vi "MTMount_logEvent_heartbeat.vi"(8 "error in (no error)":errorcluster, 11 "logevent_heartbeat_Ctl":T1) -> (0 "error out":errorcluster, 2 "function return":i32, 3 "logevent_heartbeat_Ctl out":T1)   [LabVIEW 2018, in "SALLV_MTMount.lvlib"]
doc: "int MTMount_shm_logEvent_heartbeatLV(MTMount_logevent_heartbeatLV *logevent_heartbeat_Ctl );"
uses:
  SALLV_MTMount.lvlib
  DataTypes/logevent_heartbeat.ctl
  SALLV_MTMount.so
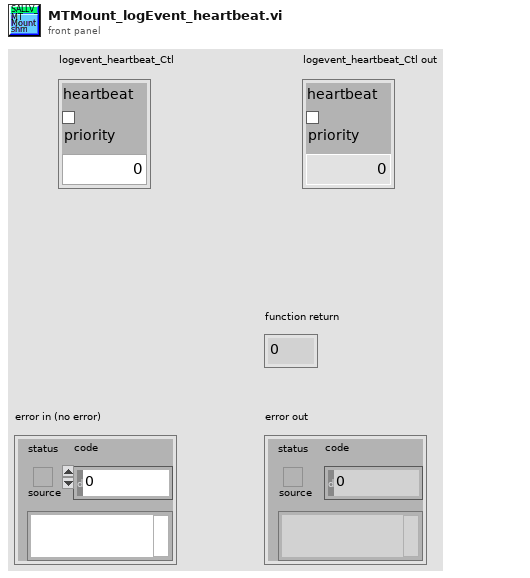
[diagram p1: front panel]
types:
  T1 = typedef "SALLV_MTMount.lvlib/logevent_heartbeat.ctl" = cluster{"heartbeat":bool, "priority":i32}
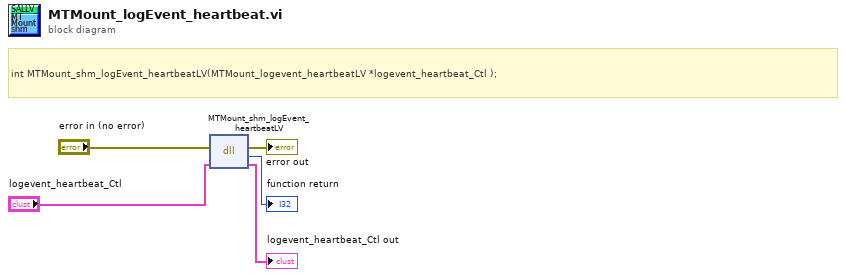
[diagram p0: block diagram]
diagram:
  # "int MTMount_shm_logEvent_heartbeatLV(MTMount_logevent_heartbeatLV *logevent_heartbeat_Ctl );"
  n1 = dll-call lib="home/ttsai/Document/salApiMTMount/SALLV_MTMount/SALLV_MTMount.*" fn="MTMount_shm_logEvent_heartbeatLV"(error in="error in (no error)", "logevent_heartbeat_Ctl"="logevent_heartbeat_Ctl") -> (error out=→"error out":errorcluster, →"function return":i32, "logevent_heartbeat_Ctl"=→"logevent_heartbeat_Ctl out":T1)  [unwired: 2 in, 1 out]
